vi "PointMeasurementStatusFCG.vi"(8 "error in":errorcluster, 9 "Set_Get":enum16{"Set", "Get"}(ring), 11 "Value":bool=TRUE) -> (0 "error out":errorcluster, 3 "Get":bool)   [LabVIEW 2011]
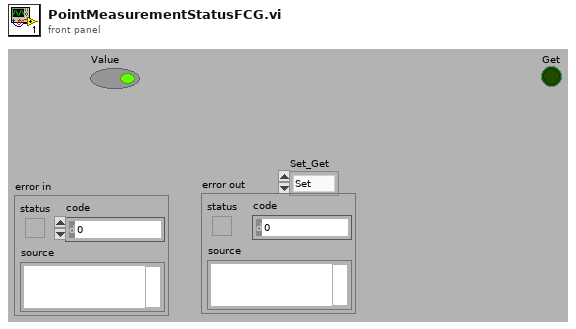
[diagram p1: front panel]
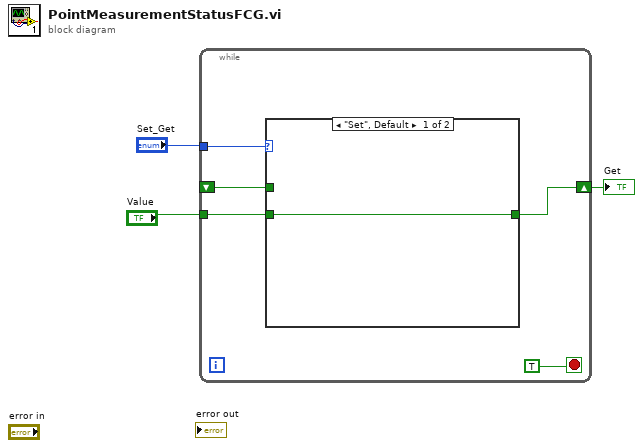
[diagram p0: block diagram]
diagram:
  n1 = while {
    tunnel: "Set_Get" -> [w8]
    tunnel: "Value" -> [w7]
    shift-right: [w6] -> w1
    shift-left: _ -> [w5]
    stop <- TRUE stop-if-true
    n2 = case shown="\"Set\", Default" w8 {
      tunnel: w7 -> [w9 _]
      tunnel: [w9 w10] -> w6
      tunnel: w5 -> [_ w10]
      frame "Set", Default {
      }
      frame "Get" {
      }
    }
  }
  "Get" <- w1
